vi "EthernetIP_CompactLogix.vi"() -> ()   [LabVIEW 2013]
uses:
  <vilib>/ethernetip/ethernetip.lvlib
  <vilib>/ethernetip/ethernetip.llb/EthernetIP Tag Write BOOL.vi
  <vilib>/ethernetip/ethernetip.llb/EthernetIP Tag Write INT.vi
  <vilib>/ethernetip/ethernetip.llb/EthernetIP Tag Read INT.vi
panel:
  out "데이터 출력 2":string
  in  "정지 버튼":bool
  out "추가된 배열":i32[](array[numeric])
  out "웨이브폼 그래프":i32[](graph)
  out "축3":u8
  out "종료루프":i32
  out "축2":u8
  out "축1":u8
  out "데이터 출력":string
  in  "Error In":errorcluster caption="에러 입력"
  out "Error Out":errorcluster caption="에러 출력"
  out "Data 2":sgl[](array[numeric])
  in  "Data":u8[](array[numeric])
  out "배열_OUT":bool[](array[boolean])
  in  "타임아웃":i32(knob)=1000 scale=0.0..1000.0
  in  "PB_TAG":bool
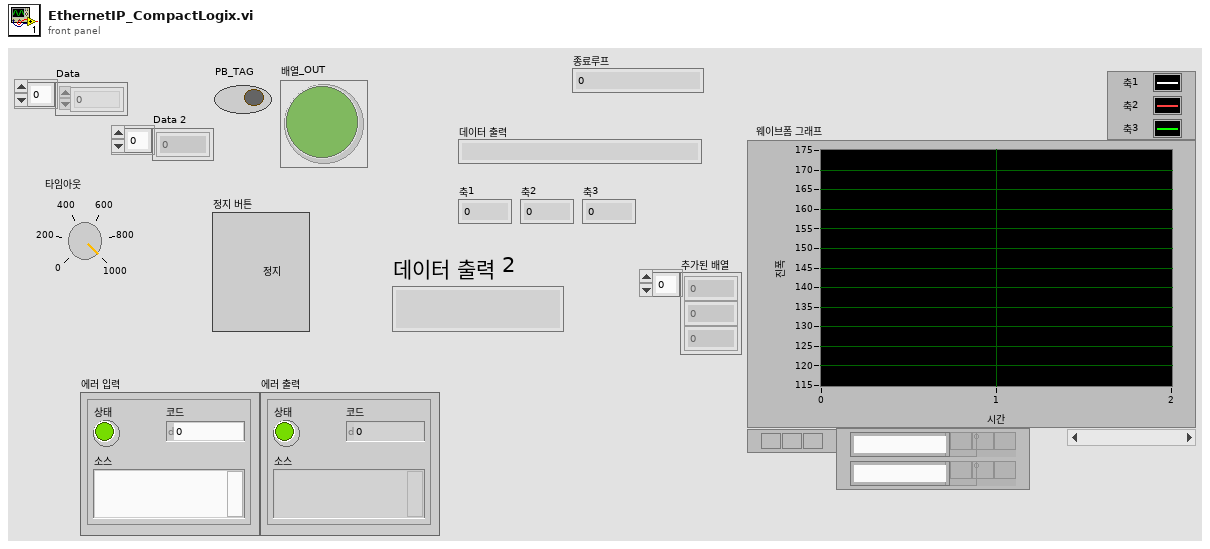
[diagram p1: front panel]
types:
  T1 = typedef "ethernetip.lvlib/ethernetip.ctl" = refnum<k21>
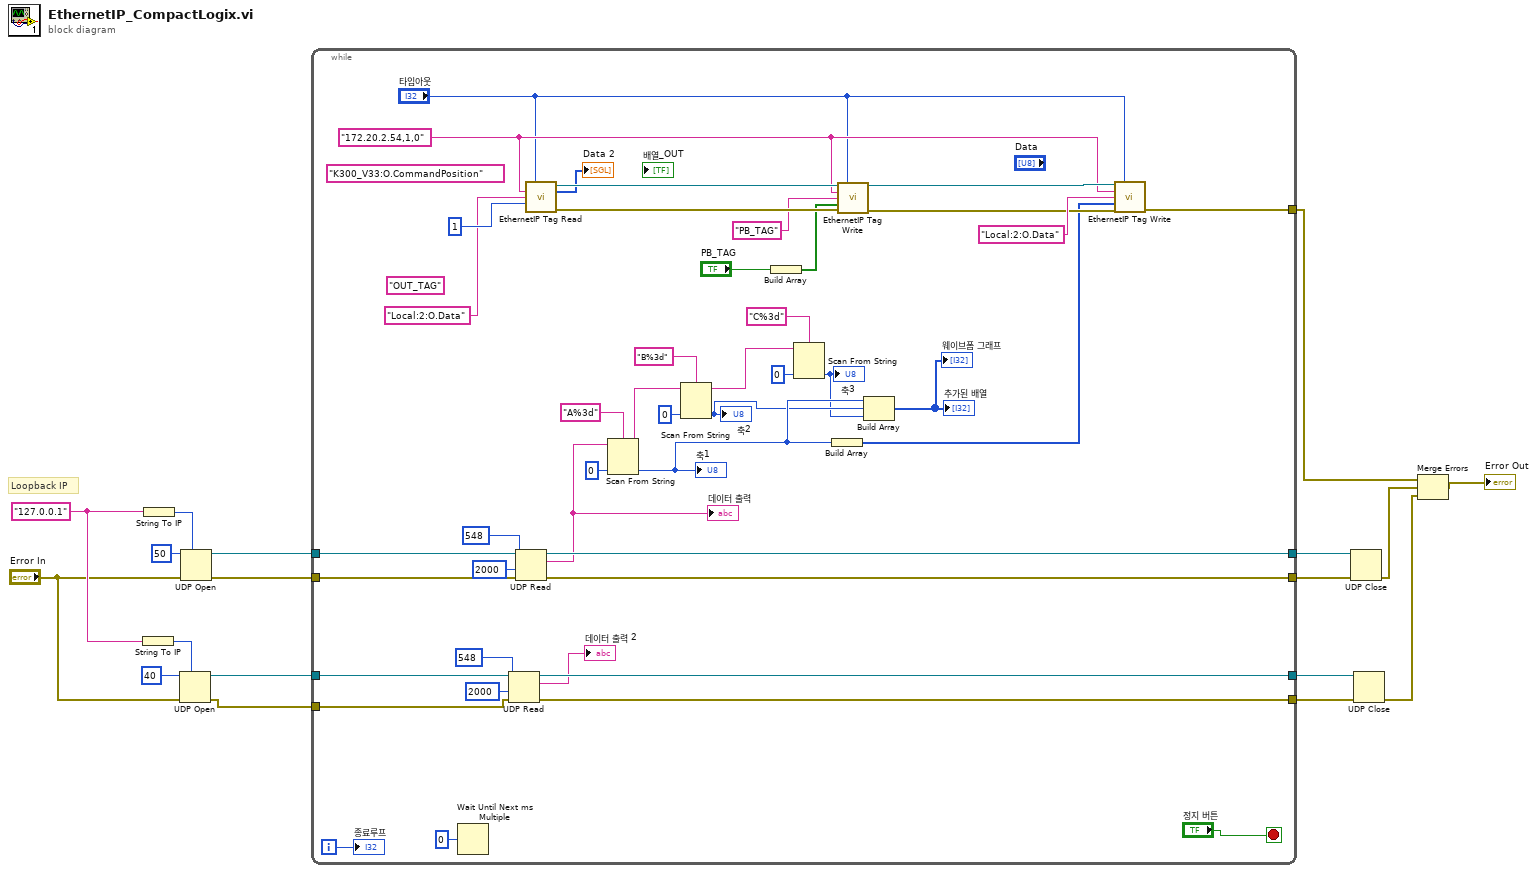
[diagram p0: block diagram]
diagram:
  w5 = "127.0.0.1"
  # "Loopback IP"
  n1 = String To IP(1:w5) -> (0:w9:u32)
  n2 = String To IP(1:w5) -> (0:w10:u32)
  n3 = UDP Open(7:w9, 8:"Error In", 11:u16 40 ("포트")) -> (port=w7:refnum<k16>, 0:w6:errorcluster)  [unwired: 2 in, 1 out]
  n4 = UDP Open(7:w10, 8:"Error In", 11:u16 50 ("포트")) -> (port=w18:refnum<k16>, 0:w16:errorcluster)  [unwired: 2 in, 1 out]
  n5 = while {
    tunnel: [w61] -> w13
    tunnel: w18 -> [w49]
    tunnel: [w48] -> w17
    tunnel: w16 -> [w47]
    tunnel: [w46] -> w15
    tunnel: w7 -> [w23]
    tunnel: w6 -> [w22]
    tunnel: [w21] -> w3
    tunnel: [w20] -> w2
    i -> [w36]
    stop <- "정지 버튼" stop-if-true
    (unwired) "K300_V33:O.CommandPosition" ("Tag Name")
    (unwired) "OUT_TAG" ("Tag Name")
    w54 = "172.20.2.54,1,0" ("Network Path")
    n6 = Wait Until Next ms Multiple(millisecond multiple=u32 0 ("ms 배수")) -> ()  [unwired: 1 out]
    n7 = UDP Read(connection ID=w23, max size (548)=548 ("최대 크기(548)"), timeout ms (25000)=2000 ("타임아웃 ms (25000)"), 8:w22) -> (data out=→"데이터 출력 2":string, error out=w20:errorcluster, 3:w21:refnum<k16>)  [unwired: 2 out]
    n8 = UDP Read(connection ID=w49, max size (548)=548 ("최대 크기(548)"), timeout ms (25000)=2000 ("타임아웃 ms (25000)"), 8:w47) -> (data out=w42:string, error out=w46:errorcluster, 3:w48:refnum<k16>)  [unwired: 2 out]
    "데이터 출력" <- w42
    n9 = call-poly <vilib>:"EthernetIP Tag Read.vi"("Timeout (ms)"="타임아웃", "Network Path"=w54, "Tag Name"="Local:2:O.Data", "Number of Elements"=u32 1) -> ("Session out"=w59:T1, "Data"=→"Data 2":i16[], "error out"=w56:errorcluster)  [unwired: 9 in]
    n10 = Scan From String(format string="A%3d" ("포맷 문자열"), input string=w42, default 1=0 ("기본값 1")) -> (remaining string=w37:string, output 1=w29:i32)  [unwired: 2 in, 2 out]
    "축1" <- w29
    n11 = Scan From String(format string="B%3d" ("포맷 문자열"), input string=w37, default 1=0 ("기본값 1")) -> (remaining string=w33:string, output 1=w28:i32)  [unwired: 2 in, 2 out]
    "축2" <- w28
    n12 = Build Array("PB_TAG") -> (w52:bool[])
    n13 = Scan From String(format string="C%3d" ("포맷 문자열"), input string=w33, default 1=0 ("기본값 1")) -> (output 1=w27:i32)  [unwired: 2 in, 3 out]
    "축3" <- w27
    n14 = Build Array(w29) -> (w31:i32[])
    n15 = call-poly <vilib>:"EthernetIP Tag Write.vi"("Session in"=w59, "Timeout (ms)"="타임아웃", "Network Path"=w54, "Tag Name"="PB_TAG", "Data"=w52, "error in"=w56) -> ("Session out"=w57:T1, "error out"=w55:errorcluster)  [unwired: 8 in]
    n16 = Build Array(w29, w28, w27) -> (→"웨이브폼 그래프" →"추가된 배열":i32[])
    n17 = call-poly <vilib>:"EthernetIP Tag Write.vi"("Session in"=w57, "Timeout (ms)"="타임아웃", "Network Path"=w54, "Tag Name"="Local:2:O.Data", "Data"=w31, "error in"=w55) -> ("error out"=w61:errorcluster)  [unwired: 8 in, 1 out]
    "종료루프" <- w36
  }
  n18 = UDP Close(connection ID=w17, 8:w15) -> (error out=w14:errorcluster)  [unwired: 1 out]
  n19 = UDP Close(connection ID=w3, 8:w2) -> (error out=w1:errorcluster)  [unwired: 1 out]
  n20 = Merge Errors(w13, w14, w1) -> (→"Error Out":errorcluster)
